vi "Data Scaling.vi"(0 "Logging queue element in":T1={"Imaging Protocol"=enum."Live Imaging", "Number of Trials"=0, "Frame Size"=512, "# Averaged frames"=0, "Dwell time (us)"=0.0, "Index of Z-plane"=0, "Timelapse?"=FALSE, "Logging process is active"=FALSE, "Speed logging enabled"=FALSE, "tdms file ref"=refnum, "path"=path "", "Trial Number"=0, "Expected # points acquired"=FALSE, "Manually stopped"=FALSE, "Last trial"=FALSE, "Ch0 data"=[], "Ch1 data"=[], "Image Time"=[], "Continuous Time"=[], "Points acquired"={"Ch0 last trial"=0, "Ch1 last trial"=0, "All trials"=0}, "HW Timings File"=refnum} {"Frame Size" items=["100X100"=100, "128X128"=128, "200X200"=200, "256X256"=256, "512X512"=512, "1024x1024"=1024, "2048x2048"=2048]; "Dwell time (us)" format="%#.6g"}, 11 "error in":errorcluster) -> (8 "Two channel data":dbl[][](array[numeric]), 15 "error out":errorcluster)   [LabVIEW 2017]
uses:
  Typedefs/Logging queue element.ctl
  Typedefs/Imaging Protocols enum.ctl
  Typedefs/Frame Size.ctl
  Typedefs/Acquired points count.ctl
panel:
  out "size(s)":i32
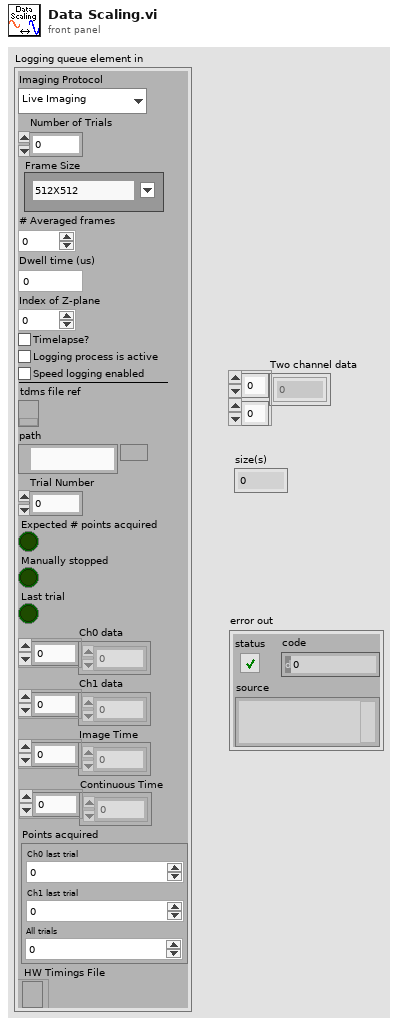
[diagram p1: front panel]
types:
  T1 = typedef "Logging queue element.ctl" = cluster{"Imaging Protocol":T2, "Number of Trials":u16, "Frame Size":T3, "# Averaged frames":u16, "Dwell time (us)":dbl, "Index of Z-plane":i32, "Timelapse?":bool, "Logging process is active":bool, "Speed logging enabled":bool, "tdms file ref":refnum<k34>, "path":path, "Trial Number":i32, "Expected # points acquired":bool, "Manually stopped":bool, "Last trial":bool, "Ch0 data":u32[], "Ch1 data":u32[], "Image Time":u64[], "Continuous Time":u64[], "Points acquired":T4, "HW Timings File":refnum<file>}
  T2 = typedef "Imaging Protocols enum.ctl" = enum16{"AOL Z-Stack", "Motor Z Stack", "Functional Acquisition", "Single Plane Acquisition", "Volume Acquisition", "Live Imaging", "Live Plane Imaging", "Live Volume Imaging"}
  T3 = typedef "Frame Size.ctl" = u16
  T4 = typedef "Acquired points count.ctl" = cluster{"Ch0 last trial":u64, "Ch1 last trial":u64, "All trials":u64}
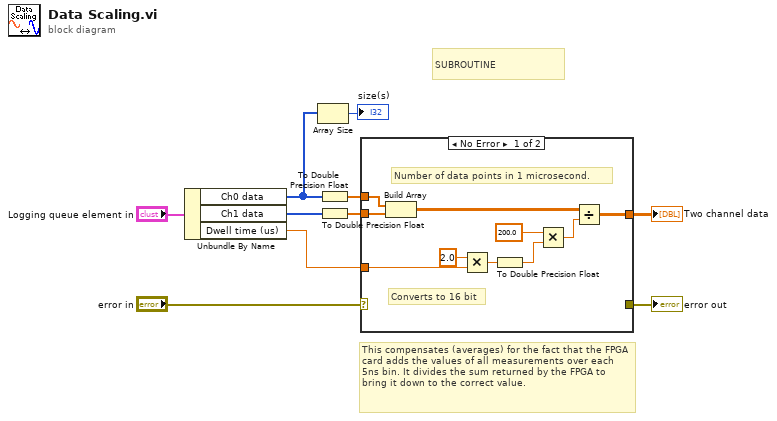
[diagram p0: block diagram]
diagram:
  # "SUBROUTINE"
  # "This compensates (averages) for the fact that the FPGA card adds the values of all measurements over each 5ns bin. It divides the sum returned by the FPGA to bring it down to the correct value."
  n1 = Unbundle By Name("Logging queue element in") -> ("Ch0 data"=w3:u32[], "Ch1 data"=w5:u32[], "Dwell time (us)"=w1:dbl)
  n2 = Array Size(array=w3) -> (size(s)=→"size(s)":i32)
  n3 = To Double Precision Float(number=w3) -> (double precision float=w6:dbl[])
  n4 = To Double Precision Float(number=w5) -> (double precision float=w4:dbl[])
  n5 = case shown="No Error" "error in" {
    selector: "error in" -> [_ w21]
    tunnel: [_ w21] -> w9
    tunnel: w6 -> [w17 _]
    tunnel: [w19 _] -> w7
    tunnel: w1 -> [w20 _]
    tunnel: w4 -> [w18 _]
    frame No Error {
      # "Number of data points in 1 microsecond."
      # "Converts to 16 bit"
      n6 = Build Array(w17, w18) -> (w16:dbl[][])
      n7 = Multiply(x=2.0, y=w20) -> (x*y=w14:dbl)
      n8 = To Double Precision Float(number=w14) -> (double precision float=w13:dbl)
      n9 = Multiply(x=200.0, y=w13) -> (x*y=w11:dbl)
      n10 = Divide(x=w16, y=w11) -> (x/y=w19:dbl[][])
    }
    frame Error {
    }
  }
  "error out" <- w9
  "Two channel data" <- w7
